vi "List controls.vi"(8 "error in (no error)":errorcluster, 11 "SettingsFileIQpid in":refnum<class "SettingsFileIQpid.lvclass">) -> (0 "error out":errorcluster, 2 "Control names":string[](array[string]), 3 "SettingsFileIQpid out":refnum<class "SettingsFileIQpid.lvclass">)   [LabVIEW 2018, in "SettingsFileIQpid.lvclass"]
uses:
  SettingsFileIQpid.lvclass
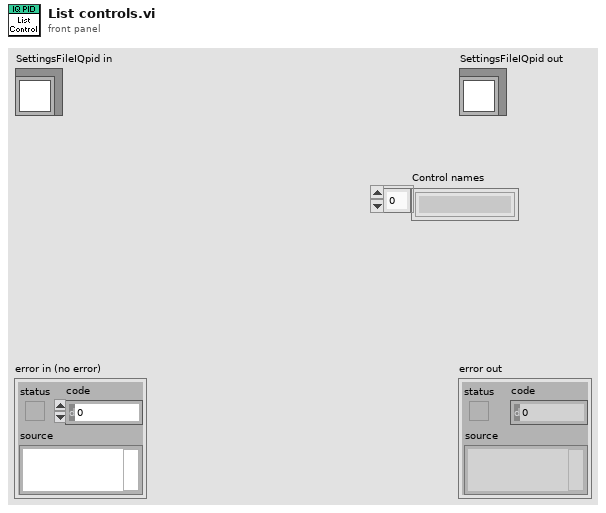
[diagram p1: front panel]
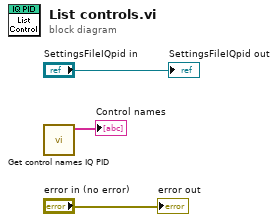
[diagram p0: block diagram]
diagram:
  n1 = call "Get control names IQ PID.vi"() -> ("Names"=→"Control names":string[])  [unwired: 11 in]
  "error out" <- "error in (no error)"
  "SettingsFileIQpid out" <- "SettingsFileIQpid in"
